vi "CreateIterator.vi"(0 "object in":refnum<class "Tree.lvclass">, 2 "TraversalType":T1, 5 "Error In":errorcluster) -> (14 "object out":refnum<class "Tree.lvclass">, 16 "Iterator":refnum<class "Iterator.lvclass">, 19 "Error Out":errorcluster)   [LabVIEW 2024, in "Tree.lvclass"]
uses:
  Tree.lvclass
  Iterator_interface/Iterator.lvclass
  BFSIterator_class/BFSTreeIterator.lvclass
  C:/Users/burakkorkmaz/Desktop/Leveling/labview-desing-patterns/Iterator Pattern/Iterator_interface/Iterator.lvclass
  DFSIterator_class/DFSTreeIterator.lvclass
  Tree.lvclass/Tree.ctl
  C:/Users/burakkorkmaz/Desktop/Leveling/labview-desing-patterns/Iterator Pattern/BFSIterator_class/BFSTreeIterator.lvclass
  C:/Users/burakkorkmaz/Desktop/Leveling/labview-desing-patterns/Iterator Pattern/DFSIterator_class/DFSTreeIterator.lvclass
  Support/Traversal Type.ctl
panel:
  # "Connector Pane"
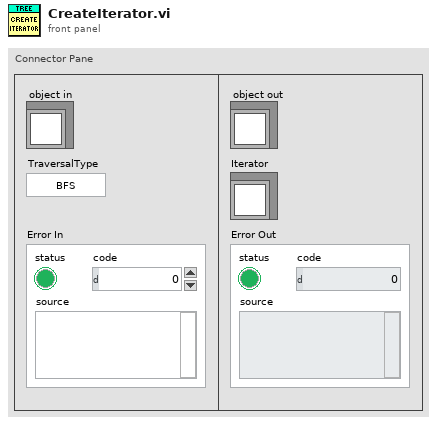
[diagram p1: front panel]
types:
  T1 = typedef "Traversal Type.ctl" = enum16{"BFS", "DFS"}
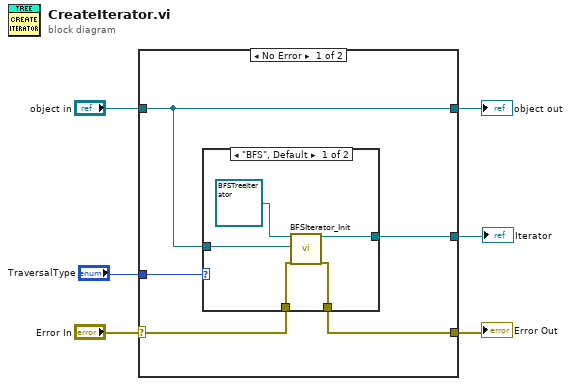
[diagram p0: block diagram]
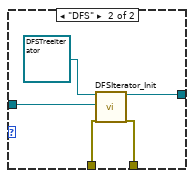
[diagram p2: hidden frame]
diagram:
  n1 = case shown="No Error" "Error In" {
    selector: "Error In" -> [w11 w23]
    tunnel: [w10 w23] -> w5
    tunnel: [w8 w22] -> w3
    tunnel: "object in" -> [w8 w22]
    tunnel: [w9 _] -> w2
    tunnel: "TraversalType" -> [w7 _]
    frame No Error {
      n2 = case shown="\"BFS\", Default" w7 {
        tunnel: w11 -> [w14 w21]
        tunnel: [w13 w20] -> w10
        tunnel: [w12 w19] -> w9
        tunnel: w8 -> [w16 w17]
        frame "BFS", Default {
          n3 = call "BFSIterator_Init.vi"("object in"=refnum<class "BFSTreeIterator.lvclass"> refnum ("BFSIterator"), "ItearableCollection"=w16, "Error In"=w14) -> ("object out"=w12:refnum<class "BFSTreeIterator.lvclass">, "Error Out"=w13:errorcluster)  [unwired: 15 in]
        }
        frame "DFS" {
          n4 = call "DFSIterator_Init.vi"("object in"=refnum<class "DFSTreeIterator.lvclass"> refnum ("DFSIterator"), "ItearableCollection"=w17, "Error In"=w21) -> ("object out"=w19:refnum<class "DFSTreeIterator.lvclass">, "Error Out"=w20:errorcluster)  [unwired: 15 in]
        }
      }
    }
    frame Error {
    }
  }
  "Error Out" <- w5
  "object out" <- w3
  "Iterator" <- w2
